vi "svx_Orbit Update Data.vi"(6 "State in":T1={"X Scale"={"Name"="Horizontal", "FString"="%#.2g", "Major Color"=16777238, "Minor Color"=16777216, "Scale Visible"=TRUE, " Label Visible"=TRUE, "Grid Style"=1}, "Y Scale"={"Name"="Vertical", "FString"="%#.2g", "Major Color"=16777238, "Minor Color"=16777216, "Scale Visible"=TRUE, " Label Visible"=TRUE, "Grid Style"=1}, "Plot"={"Point Style"=0, "Line Width"=0, "Line Style"=0, "Plot Color"=9727, "Point/fill"=0}, "Arrow/Crosshair Color"=9727, "Tacho Point Color"=16711680, "Container Bounds"={"Width"=563, "Height"=294}, "Axis Maximum"=10.0, "Probe Angles"={"Angle X"=0.0, "Angle Y"=1.5707963267948966}, "Background Color"=16777226, "Cursor"={"Cursor Point Style"=13, "Cursor Style"=4, "Cursor Line Width"=1, "Cursor Line Style"=0, "Cursor Color"=9727, "Cursor Name Visible"=TRUE, "Cursor Visible"=TRUE, "Cursor Position"={"X"=0.0, "Y"=0.0}, "Cursor Index"=0, "Cursor Lock"=FALSE}, "Elliptical Info"=[], "Legend Visible"=TRUE, "Scale Range Change"=refnum, "Strings[]"={"Custom pair name"=FALSE, "Row Strings []"=[], "Column Strings []"=[]}, "Index"=[{"pair index"=0, "order index"=0}], " Parents Tags"=[], "Children Tags"=[], "Open?"=[], "Label"="", "Legend Width"=120, "Pair Strings Changed?"=FALSE, "Size"=[], "Legend Background"=16777226, "Legend Font"=16777222, "Cursor Release"=refnum, "Autoscale"=TRUE, "Precession Direction"=[], "Item Width"=0, "User Pair Strings []"=[], "Users Order Strings []"=[], "Autoscale Once"=TRUE, "Property Write"=refnum} caption="State" {"Index"."order index" min=0; "Index"."pair index" min=0; "Axis Maximum" min=0.0}, 7 "orbit plot":T3, 11 "Orbit Plot":refnum<vi>) -> (4 "State out":T1={"X Scale"={"Name"="Horizontal", "FString"="%#.2g", "Major Color"=16777238, "Minor Color"=16777216, "Scale Visible"=TRUE, " Label Visible"=TRUE, "Grid Style"=1}, "Y Scale"={"Name"="Vertical", "FString"="%#.2g", "Major Color"=16777238, "Minor Color"=16777216, "Scale Visible"=TRUE, " Label Visible"=TRUE, "Grid Style"=1}, "Plot"={"Point Style"=0, "Line Width"=0, "Line Style"=0, "Plot Color"=9727, "Point/fill"=0}, "Arrow/Crosshair Color"=9727, "Tacho Point Color"=16711680, "Container Bounds"={"Width"=563, "Height"=294}, "Axis Maximum"=10.0, "Probe Angles"={"Angle X"=0.0, "Angle Y"=1.5707963267948966}, "Background Color"=16777226, "Cursor"={"Cursor Point Style"=13, "Cursor Style"=4, "Cursor Line Width"=1, "Cursor Line Style"=0, "Cursor Color"=9727, "Cursor Name Visible"=TRUE, "Cursor Visible"=TRUE, "Cursor Position"={"X"=0.0, "Y"=0.0}, "Cursor Index"=0, "Cursor Lock"=FALSE}, "Elliptical Info"=[], "Legend Visible"=TRUE, "Scale Range Change"=refnum, "Strings[]"={"Custom pair name"=FALSE, "Row Strings []"=[], "Column Strings []"=[]}, "Index"=[{"pair index"=0, "order index"=0}], " Parents Tags"=[], "Children Tags"=[], "Open?"=[], "Label"="", "Legend Width"=120, "Pair Strings Changed?"=FALSE, "Size"=[], "Legend Background"=16777226, "Legend Font"=16777222, "Cursor Release"=refnum, "Autoscale"=TRUE, "Precession Direction"=[], "Item Width"=0, "User Pair Strings []"=[], "Users Order Strings []"=[], "Autoscale Once"=TRUE, "Property Write"=refnum} caption="State" {"Index"."order index" min=0; "Index"."pair index" min=0; "Axis Maximum" min=0.0})   [LabVIEW 2017, in "SVX Orbit.xctl"]
uses:
  <vilib>/addons/_XControls/Orbit Plot/SVX Orbit.xctl
  <vilib>/addons/_XControls/Orbit Plot/subVIs/svx_Orbit Data.ctl
  <vilib>/addons/_XControls/Orbit Plot/subVIs/svx_Orbit Internal State.ctl
  <vilib>/addons/_XControls/Orbit Plot/subVIs/svx_Orbit Bounds.ctl
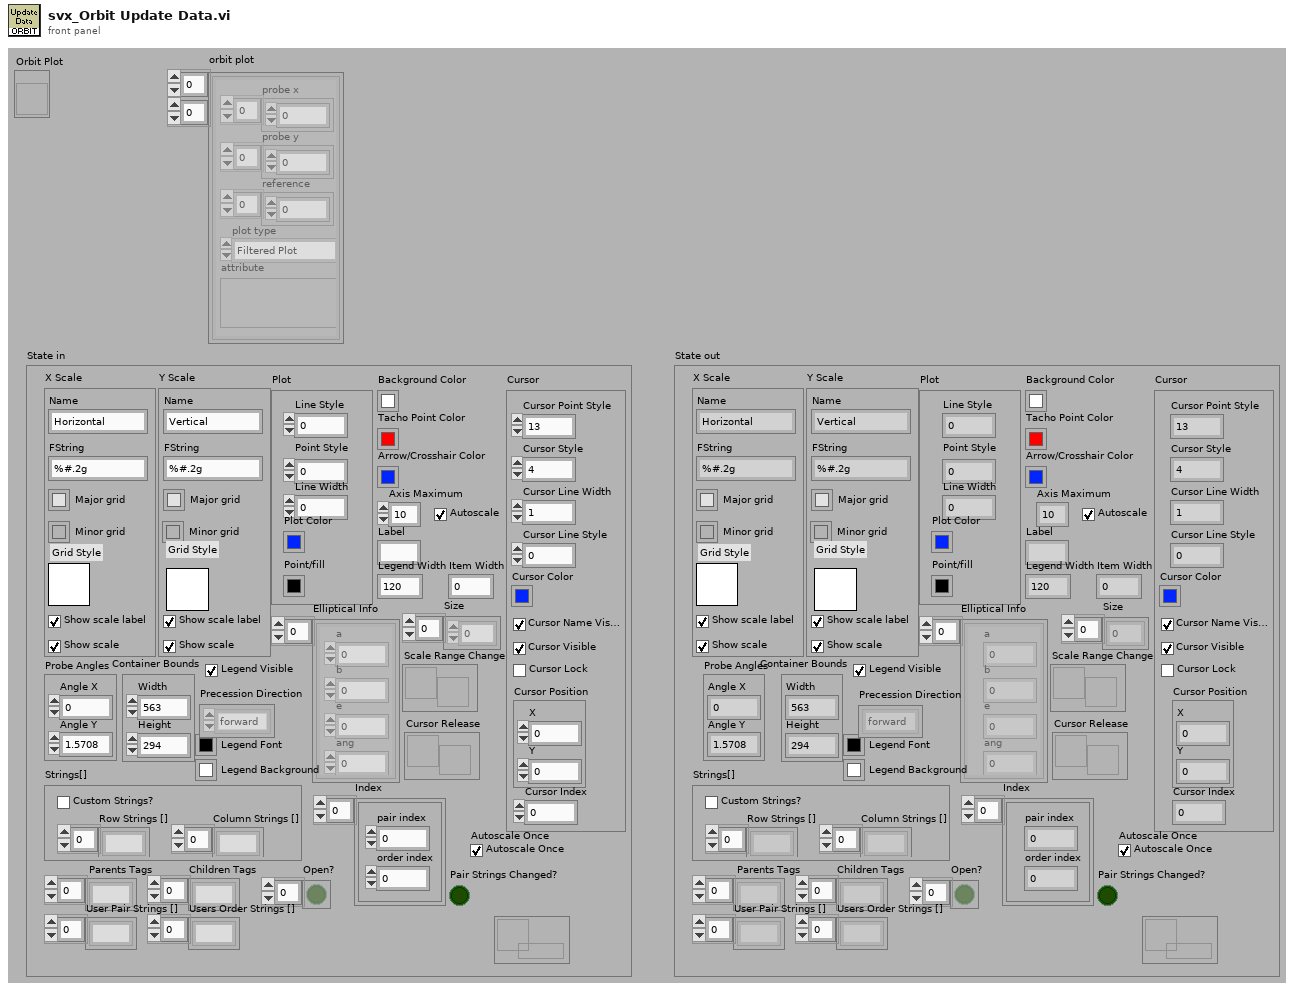
[diagram p1: front panel]
types:
  T1 = typedef "SVX Orbit.xctl/svx_Orbit Internal State.ctl" = cluster{"X Scale":cluster{"Name":string, "FString":string, "Major Color":u32, "Minor Color":u32, "Scale Visible":bool, " Label Visible":bool, "Grid Style":u16}, "Y Scale":cluster{"Name":string, "FString":string, "Major Color":u32, "Minor Color":u32, "Scale Visible":bool, " Label Visible":bool, "Grid Style":u16}, "Plot":cluster{"Point Style":u8, "Line Width":u8, "Line Style":u8, "Plot Color":u32, "Point/fill":u32}, "Arrow/Crosshair Color":u32, "Tacho Point Color":u32, "Container Bounds":T2, "Axis Maximum":dbl, "Probe Angles":cluster{"Angle X":dbl, "Angle Y":dbl}, "Background Color":u32, "Cursor":cluster{"Cursor Point Style":u8, "Cursor Style":u8, "Cursor Line Width":u8, "Cursor Line Style":u8, "Cursor Color":u32, "Cursor Name Visible":bool, "Cursor Visible":bool, "Cursor Position":cluster{"X":dbl, "Y":dbl}, "Cursor Index":i32, "Cursor Lock":bool}, "Elliptical Info":cluster{"a":dbl, "b":dbl, "e":dbl, "ang":dbl}[], "Legend Visible":bool, "Scale Range Change":refnum<user-event>, "Strings[]":cluster{"Custom pair name":bool, "Row Strings []":string[], "Column Strings []":string[]}, "Index":cluster{"pair index":i32, "order index":i32}[], " Parents Tags":string[], "Children Tags":string[], "Open?":bool[], "Label":string, "Legend Width":u32, "Pair Strings Changed?":bool, "Size":i32[], "Legend Background":u32, "Legend Font":u32, "Cursor Release":refnum<user-event>, "Autoscale":bool, "Precession Direction":enum16{"forward", "backward"}[], "Item Width":u32, "User Pair Strings []":string[], "Users Order Strings []":string[], "Autoscale Once":bool, "Property Write":refnum<queue>}
  T2 = typedef "SVX Orbit.xctl/svx_Orbit Bounds.ctl" = cluster{"Width":u32, "Height":u32}
  T3 = typedef "SVX Orbit.xctl/svx_Orbit Data.ctl" = cluster{"probe x":dbl[], "probe y":dbl[], "reference":dbl[], "plot type":enum16{"Filtered Plot", "Unfiltered Plot"}, "attribute":variant}[][]
  T4 = cluster{"orbit plot X":dbl[], "orbit plot Y":dbl[]}[]
  T5 = cluster{"probe x":dbl[], "probe y":dbl[], "reference":dbl[], "plot type":enum16{"Filtered Plot", "Unfiltered Plot"}, "attribute":variant}
  T6 = cluster{"orbit plot X":dbl[], "orbit plot Y":dbl[]}
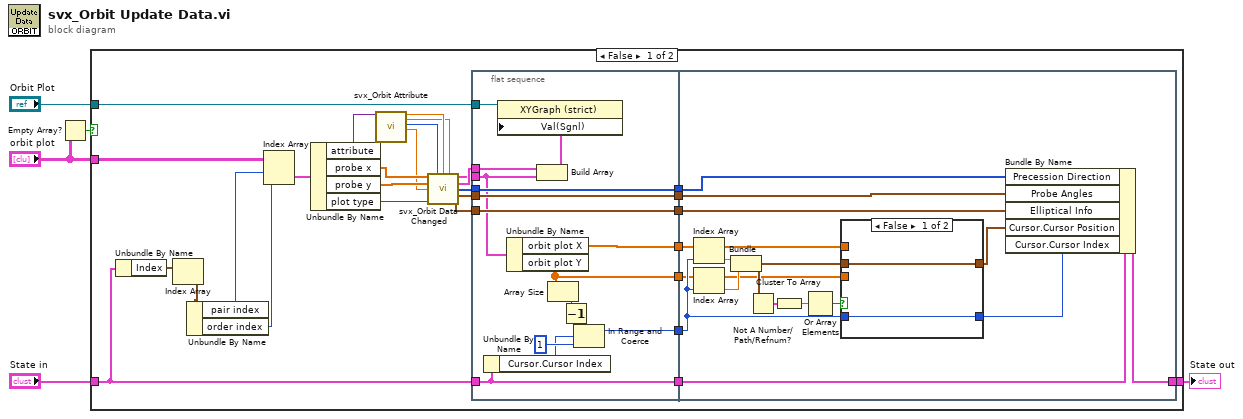
[diagram p0: block diagram]
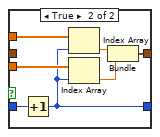
[diagram p2: hidden frame]
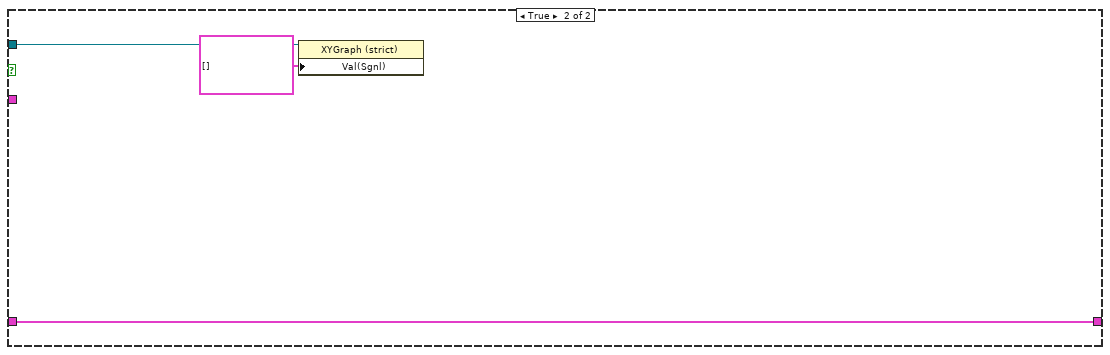
[diagram p3: hidden frame]
diagram:
  n1 = Empty Array?(array="orbit plot") -> (empty?=w1:bool)
  n2 = case shown="False" w1 {
    tunnel: "Orbit Plot" -> [w19 w76]
    tunnel: "State in" -> [w12 w77]
    tunnel: [w7 w77] -> w3
    tunnel: "orbit plot" -> [w15 _]
    frame False {
      n3 = Unbundle By Name(w12) -> ("Index"=w13:cluster{"pair index":i32, "order index":i32}[])
      n4 = Index Array(array=w13) -> (element=w14:cluster{"pair index":i32, "order index":i32})  [unwired: 1 in]
      n5 = Unbundle By Name(w14) -> ("pair index"=w11:i32, "order index"=w10:i32)
      n6 = Index Array(array=w15, index (row)=w11, index (col)=w10) -> (element=w23:T5)
      n7 = Unbundle By Name(w23) -> ("attribute"=w22:variant, "probe x"=w30:dbl[], "probe y"=w29:dbl[], "plot type"=w24:enum16{"Filtered Plot", "Unfiltered Plot"})
      n8 = call <vilib>:"svx_Orbit Attribute.vi"("attribute"=w22) -> ("probe angle X"=w28:dbl, "probe angle Y"=w27:dbl, "rotating direction"=w26:u16, "samples/rev"=w25:dbl)  [unwired: 13 in, 2 out]
      n9 = call <vilib>:"svx_Orbit Data Changed.vi"("orbit plot X"=w30, "shaft rotating direction"=w26, "probe angles X"=w28, "probe angles Y"=w27, "orbit plot Y"=w29, "actual samples/rev"=w25, "plot type"=w24) -> ("orbit data"=w20:T6, "tacho points"=w21:cluster{dbl[], dbl[]}, "precession direction"=w18:u16[], "probe angles"=w17:cluster{"angles X":dbl, "angles Y":dbl}, "elliptical info"=w16:cluster{"a":dbl, "b":dbl, "e":dbl, "ang":dbl}[])  [unwired: 4 in]
      n10 = flat-sequence {
        tunnel: w21 -> [w35]
        tunnel: w20 -> [w36]
        tunnel: w19 -> [w49]
        tunnel: [w44] -> w34
        tunnel: w12 -> [w44]
        tunnel: [w47] -> w33
        tunnel: w18 -> [w47]
        tunnel: [w46] -> w32
        tunnel: w17 -> [w46]
        tunnel: [w45] -> w31
        tunnel: w16 -> [w45]
        tunnel: [w43] -> w9
        tunnel: [w41] -> w8
        tunnel: [w39] -> w6
        tunnel: w34 -> [w65]
        tunnel: w33 -> [w63]
        tunnel: w32 -> [w60]
        tunnel: w31 -> [w64]
        tunnel: w6 -> [w56]
        tunnel: w9 -> [w55]
        tunnel: w8 -> [w51]
        tunnel: [w52] -> w7
        frame #0 {
          n11 = Unbundle By Name(w44) -> ("Cursor.Cursor Index"=w40:i32)
          n12 = Unbundle By Name(w36) -> ("orbit plot X"=w43:dbl[], "orbit plot Y"=w41:dbl[])
          n13 = Build Array(w35, w36) -> (w48:T4)
          n14 = property on="Property Node" class="XYGraph (strict)"(reference=w49, "Val(Sgnl)"=w48) -> ()  [unwired: 1 in, 2 out]
          n15 = Array Size(array=w41) -> (size(s)=w38:i32)
          n16 = Decrement(x=w38) -> (x-1=w37:i32)
          n17 = In Range and Coerce(upper limit=w37, x=w40, lower limit=1) -> (coerced(x)=w39:i32)  [unwired: 1 out]
        }
        frame #1 {
          n18 = Index Array(array=w55, index=w56) -> (element=w62:dbl)
          n19 = Index Array(array=w51, index=w56) -> (element=w61:dbl)
          n20 = Bundle(w62, w61) -> (w53:cluster{dbl, dbl})  [unwired: 1 in]
          n21 = Not A Number/Path/Refnum?(number/path/refnum=w53) -> (NaN/Path/Refnum?=w58:cluster{bool, bool})
          n22 = Cluster To Array(cluster=w58) -> (array=w59:bool[])
          n23 = Or Array Elements(Boolean array=w59) -> (logical OR=w57:bool)
          n24 = case shown="False" w57 {
            tunnel: w56 -> [w66 w69]
            tunnel: w55 -> [_ w73]
            tunnel: w51 -> [_ w72]
            tunnel: [w67 w70] -> w54
            tunnel: w53 -> [w67 _]
            tunnel: [w66 w68] -> w50
            frame False {
            }
            frame True {
              n25 = Increment(x=w69) -> (x+1=w68:i32)
              n26 = Index Array(array=w73, index=w68) -> (element=w74:dbl)
              n27 = Index Array(array=w72, index=w68) -> (element=w71:dbl)
              n28 = Bundle(w74, w71) -> (w70:cluster{dbl, dbl})  [unwired: 1 in]
            }
          }
          n29 = Bundle By Name(cluster=w65, "Precession Direction"=w63, "Probe Angles"=w60, "Elliptical Info"=w64, "Cursor.Cursor Position"=w54, "Cursor.Cursor Index"=w50) -> (w52:T1)
        }
      }
    }
    frame True {
      n30 = property on="Property Node" class="XYGraph (strict)"(reference=w76, "Val(Sgnl)"=T4 [] ("Value (Signaling)")) -> ()  [unwired: 1 in, 2 out]
    }
  }
  "State out" <- w3
